vi "FPGAHoppingSimulator.vi"() -> ()   [LabVIEW 2014]
uses:
  <vilib>/rvi/Emulation/niFpgaGetClockAttributes.vi
  <vilib>/rvi/Emulation/niFpgaSctlEmulationGetInTimedLoop.vi
  <vilib>/rvi/Emulation/niFpgaEmulationReportErrorSimple.vi
  <vilib>/rvi/Emulation/niFpgaCriticalErrorInLSC.vi
  <vilib>/rvi/interface/RandomDataEmulation/niFpgaRandomDataHandleErrors.vi
  <vilib>/rvi/DataTransferAndStorage/Container/Common/niFpgaContainerExecOnDevCompGetState.vi
  <vilib>/rvi/Emulation/niFpgaEmulationIsFPGAContextNoSignature.vi
  <vilib>/rvi/errors/niFpgaSetErrorForExecOnDevCompSimple.vi
  <vilib>/rvi/eio/common/nirviEmuReportErrorAndStop.vi
  <vilib>/rvi/DataTransferAndStorage/Container/Common/niFpgaContainerGetUniqueNameForEmu.vi
  <vilib>/rvi/FIFO/Fifo_Resource/nirvififoEmulationSetSize.vi
  <vilib>/rvi/FIFO/Fifo_Resource/nirviFifoEmulationQueueMgr.vi
  <instcachedir>/0/nirviFifoEmulationQueueMgr_E5CAEC123FF24DC58D834DCA3CDAA9B5.lvgen/nirviFifoEmulationQueueMgr_E5CAEC123FF24DC58D834DCA3CDAA9B5_001.vi
  <vilib>/rvi/FIFO/Fifo_Resource/nirvififoEmulationDetermineInputValidOut.vi
  <vilib>/rvi/FIFO/Fifo_Resource/nirvififoEmulationCreateLock.vi
  <vilib>/rvi/Emulation/niFpgaProcessEmulError.vi
  <vilib>/rvi/FIFO/Fifo_Resource/nirvififoEmulationObtainLock.vi
  <vilib>/rvi/FIFO/Fifo_Resource/nirvififoEmulationReleaseLock.vi
  <vilib>/rvi/occurrence/nirviWaitOnOccurrenceBase.vi
  <vilib>/rvi/errors/nirviReportUnexpectedCaseInternalError.vi
  <vilib>/rvi/errors/nirviReportUnexpectedCaseInternalError (U32).vi
  <vilib>/Utility/error.llb/Clear Errors.vi
  <vilib>/rvi/DataTransferAndStorage/Container/XNode/niFpgaContainer.xnode
  <vilib>/rvi/interface/RandomDataEmulation/nirviRandomDataFpgaReadWriteTemplate.vi
  <vilib>/rvi/FIFO/Fifo_Resource/niFpgaFifoEmulationRefIn.vi
panel:
  out "WriteNum":u32
  in  "stop":bool
  out "ZPos?":i16(graph)
  in  "Sleep":u32 caption="Count(uSec)"
  in  "BaseTime us":i16
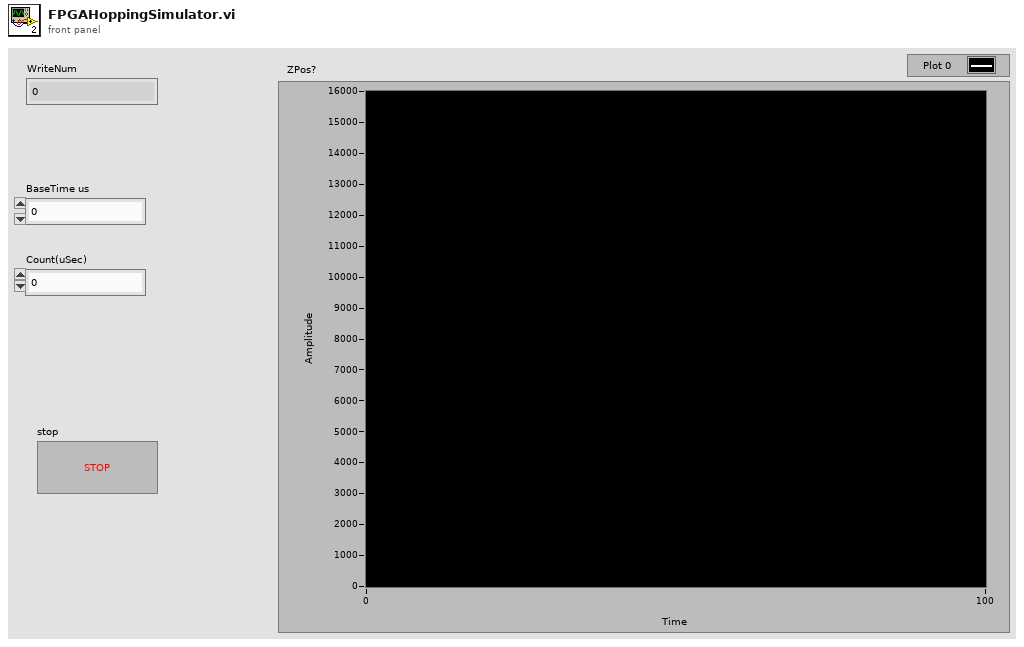
[diagram p1: front panel]
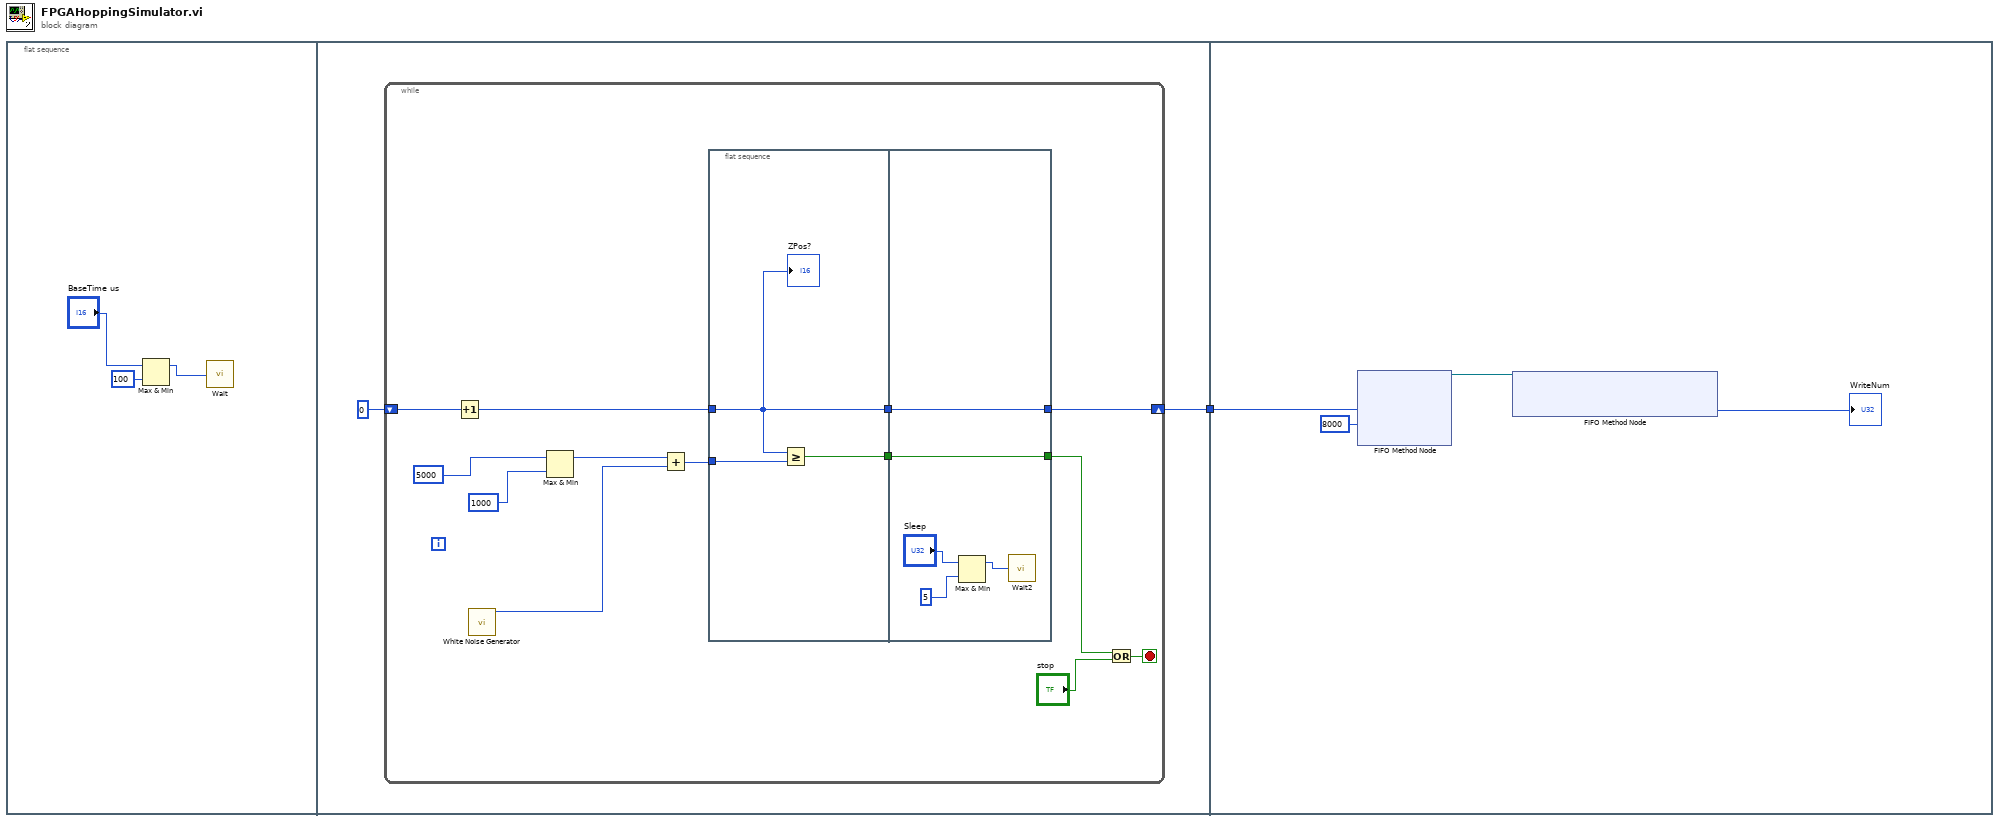
[diagram p0: block diagram]
diagram:
  n1 = flat-sequence {
    tunnel: [w5] -> w1
    tunnel: w1 -> [w31]
    frame #0 {
      n2 = Max & Min(x="BaseTime us", y=i16 100) -> (max(x,y)=w2:i16)  [unwired: 1 out]
      n3 = call "Wait"("Count(uSec)"=w2) -> ()  [unwired: 1 out]
    }
    frame #1 {
      n4 = while {
        shift-right: [w16] -> w5
        shift-left: i16 0 -> [w19]
        stop <- w11 stop-if-true
        n5 = Increment(x=w19) -> (x+1=w18:i16)
        n6 = call "White Noise Generator"() -> ("white noise out"=w7:i16)  [unwired: 15 in]
        n7 = Max & Min(x=5000, y=1000) -> (max(x,y)=w13:i32)  [unwired: 1 out]
        n8 = Add(x=w13, y=w7) -> (x+y=w14:i32)
        n9 = flat-sequence {
          tunnel: w18 -> [w20]
          tunnel: w14 -> [w22]
          tunnel: [w21] -> w17
          tunnel: [w20] -> w15
          tunnel: w17 -> [w27]
          tunnel: [w27] -> w10
          tunnel: [w23] -> w16
          tunnel: w15 -> [w23]
          frame #0 {
            n10 = Greater Or Equal?(x=w20, y=w22) -> (x >= y?=w21:bool)
            "ZPos?" <- w20
          }
          frame #1 {
            n11 = Max & Min(x="Sleep", y=u32 5) -> (max(x,y)=w26:u32)  [unwired: 1 out]
            n12 = call "Wait2"("Count(uSec)"=w26) -> ()  [unwired: 1 out]
          }
        }
        n13 = Or(x=w10, y="stop") -> (x .or. y?=w11:bool)
      }
    }
    frame #2 {
      n14 = xnode ("FIFO Method Node")("Element"=w31, "Timeout"=8000) -> ("FIFO Out"=w29:refnum<k21>)  [unwired: 1 in, 1 out]
      n15 = xnode ("FIFO Method Node")("FIFO In"=w29) -> ("Number of Elements to Write"=→"WriteNum":u32)  [unwired: 1 out]
    }
  }
